vi "Stop Core.vi"(10 "final error code":i32, 11 "Multi Instrument Handler in":refnum<class "Multi Instrument Handler.lvclass">) -> (3 "Multi Instrument Handler out":refnum<class "Multi Instrument Handler.lvclass">)   [LabVIEW 2020, in "Instrument Handler.lvlib" / "Multi Instrument Handler.lvclass"]
doc: "(<B>Filename</B>: Actor Framework.lvlib:Actor.lvclass:Stop Core.vi)\n\nDefines what the actor does before it stops. Use the <B>final error code</B> input to determine whether the actor shut down in response to an error.\n\nBy default, this method does nothing. A descendant class may override it to define behavior, such as shutting down any processes the actor initiated in its override of the Actor Core method."
uses:
  Multi Instrument Handler.lvclass
  Multi Instrument Handler.lvclass/Multi Instrument Handler.ctl
  PPL/HDH.Actor Framework.Core.Sequencer.lvlibp/Sequencer/Sequencer.lvclass
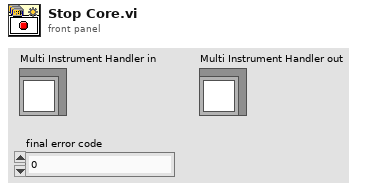
[diagram p1: front panel]
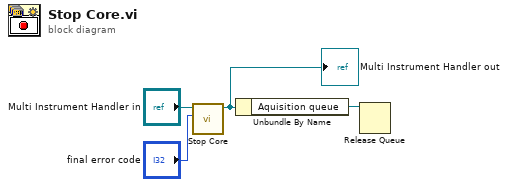
[diagram p0: block diagram]
diagram:
  n1 = call-parent "Stop Core.vi"("final error code"="final error code", "Sequencer in"="Multi Instrument Handler in") -> ("Sequencer out"=w2:refnum<class "Multi Instrument Handler.lvclass">)  [unwired: 9 in]
  "Multi Instrument Handler out" <- w2
  n2 = Unbundle By Name(w2) -> ("Aquisition queue"=w1:refnum<queue>)
  n3 = Release Queue(queue=w1) -> ()  [unwired: 2 in, 3 out]
